vi "Ltgn Cuoi Ky.vi"() -> ()   [LabVIEW 2020]
uses:
  <vilib>/MakerHub/LINX/Public/Peripherals/Analog/Analog Read 1 Chan.vi
  <vilib>/MakerHub/LINX/Public/Peripherals/Digital/Digital Write 1 Chan.vi
  <vilib>/MakerHub/LINX/Public/Peripherals/Analog/Analog Read N Chans.vi
  <vilib>/MakerHub/LINX/Public/Peripherals/Digital/Digital Write N Chans.vi
  <vilib>/MakerHub/LINX/Private/Local IO/LinxAnalogRead.vi
  <vilib>/MakerHub/LINX/Public/Utilities/Check Channel.vi
  <vilib>/MakerHub/LINX/Private/Local IO/LinxDigitalWrite.vi
  <vilib>/MakerHub/LINX/Public/Utilities/Open Serial.vi
  <vilib>/MakerHub/LINX/Private/Utilties/Generate Error.vi
  <vilib>/MakerHub/LINX/LMH-LINX.lvlib
panel:
  out "Nhiet Do":dbl
  out "V Nhiet Do":dbl
  out "LED Anh Sang":bool
  out "V quangtro":dbl
  out "Gia Tri Bien Tro":dbl
  out "V bientro":dbl
  out "LED Nhiet Do":bool
  in  "Gia tri Nguong":dbl
  out "Bieu Do Nhiet Do":dbl(graph)
  in  "Serial Port":refnum<visa-resource-name>="N/A"
  in  "stop":bool
  out "Thermometer":dbl(slide) scale=0.0..100.0
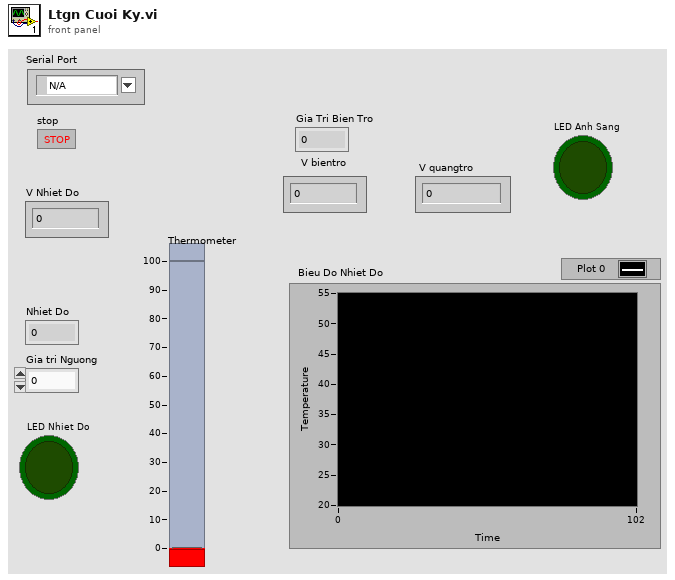
[diagram p1: front panel]
types:
  T1 = typedef "LMH-LINX.lvlib/LINX Ref.ctl" = cluster{"IO":T2, "Interface":T3, "LINX Device Config":T4}
  T2 = typedef "LMH-LINX.lvlib/Platform.ctl" = enum16{"Remote", "Local"}
  T3 = typedef "LMH-LINX.lvlib/Interface.ctl" = enum16{"Serial", "TCP"}
  T4 = typedef "LMH-LINX.lvlib/Device.lvlib/LINX Device Config.ctl" = cluster{"Interface":T3, "COM Port":refnum<visa-resource-name>, "TCP Configuration":T5, "Device Family":u8, "Device ID":u8, "Device Name":string, "TCP Ref":refnum<k5>, "Channels":T6}
  T5 = typedef "LMH-LINX.lvlib/Device.lvlib/TCP Config.ctl" = cluster{"IP Address":string, "Port":u16}
  T6 = typedef "LMH-LINX.lvlib/Channels.ctl" = cluster{"DI":u8[], "DO":u8[], "AI":u8[], "AO":u8[], "PWM":u8[], "QE":u8[], "UART":u8[], "I2C 2":u8[], "SPI":u8[], "CAN":u8[], "Servo":u8[], "AI Ref (V)":dbl, "AI Resolution (Bits)":u8, "AO Ref (V)":dbl, "AO Resolution (Bits)":u8}
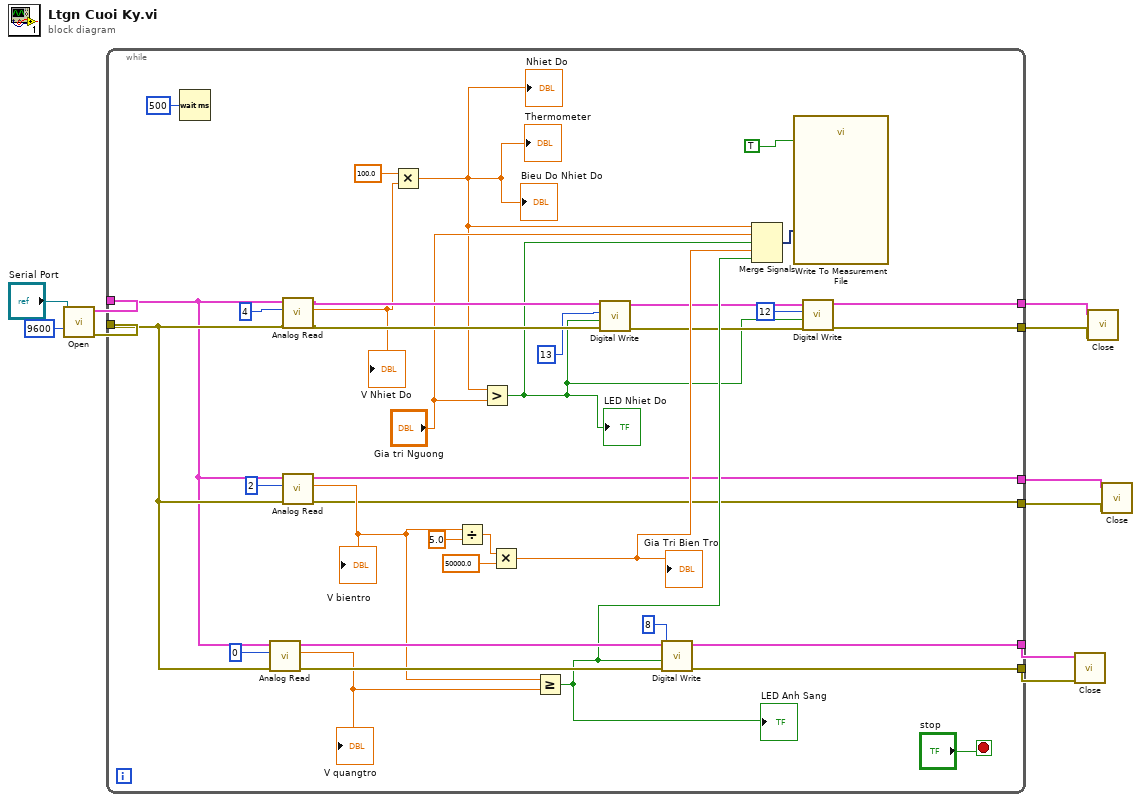
[diagram p0: block diagram]
diagram:
  n1 = call-poly <vilib>:"Open.vi"("Baud Rate Override"=u32 9600, "Serial Port"="Serial Port") -> ("Error Out"=w9:errorcluster, "LINX Resource"=w10:T1)  [unwired: 7 in, 1 out]
  n2 = while {
    tunnel: w10 -> [w19]
    tunnel: w9 -> [w20]
    tunnel: [w31] -> w2
    tunnel: [w30] -> w1
    tunnel: [w29] -> w4
    tunnel: [w28] -> w3
    tunnel: [w15] -> w6
    tunnel: [w13] -> w5
    stop <- "stop" stop-if-true
    n3 = Wait (ms)(milliseconds to wait=u32 500) -> ()  [unwired: 1 out]
    n4 = call-poly <vilib>:"Analog Read.vi"("Error In"=w20, "Analog Channel"=u8 0, "LINX Resource"=w19) -> ("Error Out"=w39:errorcluster, "Voltage"=w32:dbl, "LINX Resource"=w40:T1)  [unwired: 5 in, 1 out]
    "V quangtro" <- w32
    n5 = call-poly <vilib>:"Analog Read.vi"("Error In"=w20, "Analog Channel"=u8 4, "LINX Resource"=w19) -> ("Error Out"=w25:errorcluster, "Voltage"=w22:dbl, "LINX Resource"=w26:T1)  [unwired: 5 in, 1 out]
    "V Nhiet Do" <- w22
    n6 = call-poly <vilib>:"Analog Read.vi"("Error In"=w20, "Analog Channel"=u8 2, "LINX Resource"=w19) -> ("Error Out"=w28:errorcluster, "Voltage"=w33:dbl, "LINX Resource"=w29:T1)  [unwired: 5 in, 1 out]
    "V bientro" <- w33
    n7 = Multiply(x=100.0, y=w22) -> (x*y=w21:dbl)
    "Thermometer" <- w21
    "Bieu Do Nhiet Do" <- w21
    "Nhiet Do" <- w21
    n8 = Divide(x=w33, y=5.0) -> (x/y=w42:dbl)
    n9 = Greater?(x=w21, y="Gia tri Nguong") -> (0:w12:bool)
    "LED Nhiet Do" <- w12
    n10 = Multiply(x=w42, y=50000.0) -> (x*y=w34:dbl)
    "Gia Tri Bien Tro" <- w34
    n11 = Greater Or Equal?(x=w33, y=w32) -> (x >= y?=w35:bool)
    "LED Anh Sang" <- w35
    n12 = call-poly <vilib>:"Digital Write.vi"("Error In"=w25, "Output Value"=w12, "DO Channel"=u8 13, "LINX Resource"=w26) -> ("Error Out"=w14:errorcluster, "LINX Resource"=w16:T1)  [unwired: 6 in]
    n13 = call-poly <vilib>:"Digital Write.vi"("Error In"=w39, "Output Value"=w35, "DO Channel"=u8 8, "LINX Resource"=w40) -> ("Error Out"=w30:errorcluster, "LINX Resource"=w31:T1)  [unwired: 6 in]
    n14 = Merge Signals(w21, "Gia tri Nguong", w12, w34, w35) -> (w36:dynamicdata)
    n15 = call "Write To Measurement File"("Signals"=w36, "Enable"=TRUE) -> ()  [unwired: 15 in, 3 out]
    n16 = call-poly <vilib>:"Digital Write.vi"("Error In"=w14, "Output Value"=w12, "DO Channel"=u8 12, "LINX Resource"=w16) -> ("Error Out"=w13:errorcluster, "LINX Resource"=w15:T1)  [unwired: 6 in]
  }
  n17 = call <vilib>:"Close.vi"("Error In"=w1, "LINX Resource"=w2) -> ()  [unwired: 9 in, 1 out]
  n18 = call <vilib>:"Close.vi"("Error In"=w5, "LINX Resource"=w6) -> ()  [unwired: 9 in, 1 out]
  n19 = call <vilib>:"Close.vi"("Error In"=w3, "LINX Resource"=w4) -> ()  [unwired: 9 in, 1 out]
